vi "ARGBImageExtractRed.vi"(8 "error in (no error)":errorcluster, 10 "Greyscale Image Destination":refnum<data-value>, 11 "ARGB Image Source":refnum<data-value>) -> (0 "error out":errorcluster, 3 "Greyscale Image Destination (Duplicate)":refnum<data-value>)   [LabVIEW 2020, in "g_ar_toolkit.image.lvlib"]
uses:
  g_ar_toolkit.image.lvlib
  Extract_Options.ctl
  b49f9b5f-0d0c-44fc-96ba-8bd9d53fe8ca.vi
  <vilib>/Utility/error.llb/Error Cluster From Error Code.vi
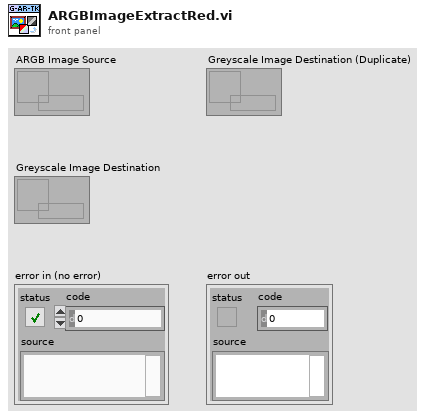
[diagram p1: front panel]
types:
  T1 = typedef "Extract_Options.ctl" = enum8{"Blue", "Green", "Red", "Alpha", "Greyscale"}
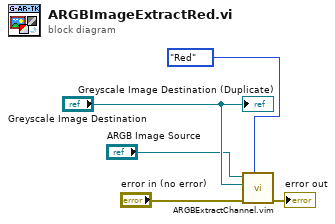
[diagram p0: block diagram]
diagram:
  n1 = call "ARGBExtractChannel.vim"("ExtractOperation"=Extract_Options."Red" ("Extract_Operation"), "error in (no error)"="error in (no error)", "Greyscale Image Destination"="Greyscale Image Destination", "ARGB Image Source"="ARGB Image Source") -> ("error out"=→"error out":errorcluster)  [unwired: 7 in]
  "Greyscale Image Destination (Duplicate)" <- "Greyscale Image Destination"
